vi "creat tasks.vi"   [LabVIEW 2017]
uses:
  <vilib>/DAQmx/create/channels.llb/DAQmx Create Channel (TEDS-AI-Current-Basic).vi
  <vilib>/DAQmx/create/channels.llb/DAQmx Create Channel (AI-Current-Basic).vi
  <resource>/objmgr/daqmx.rc
  <vilib>/DAQmx/create/channels.llb/DAQmx Create Channel (AI-Voltage-Basic).vi
  <vilib>/DAQmx/create/channels.llb/DAQmx Create Channel (AI-Temperature-RTD).vi
  <vilib>/DAQmx/create/channels.llb/DAQmx Create Channel (AI-Temperature-Thermocouple).vi
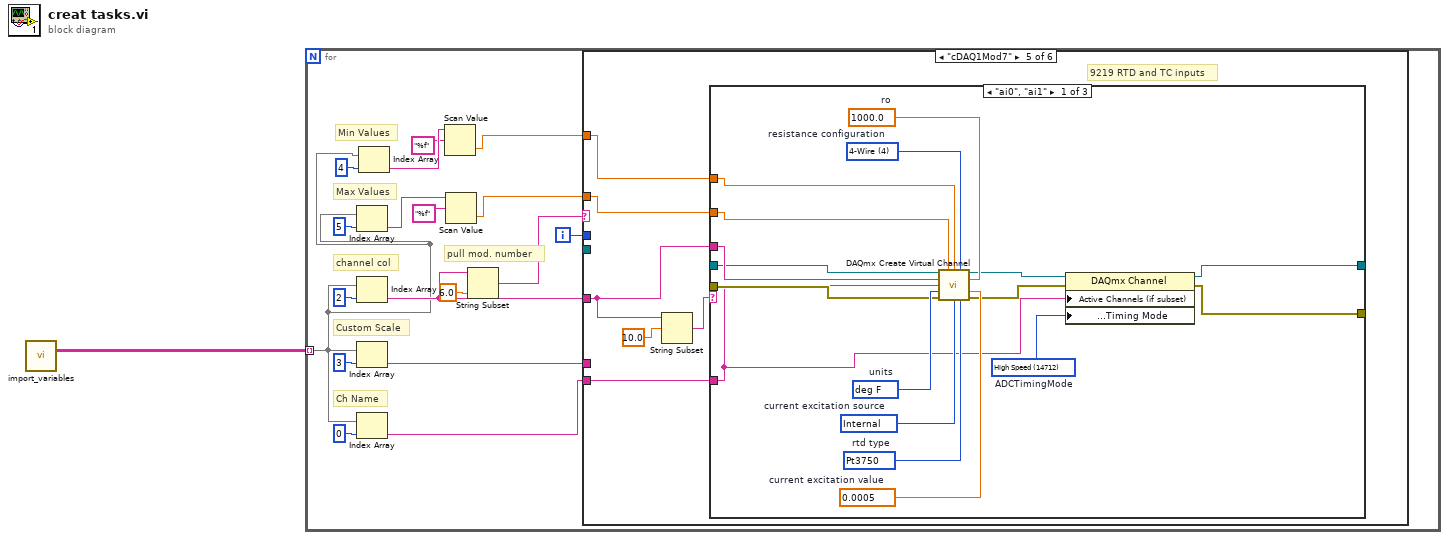
[diagram p0: block diagram]
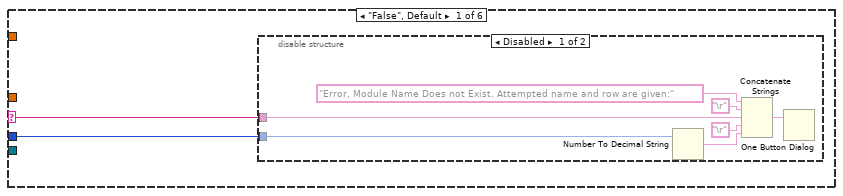
[diagram p2: hidden frame]
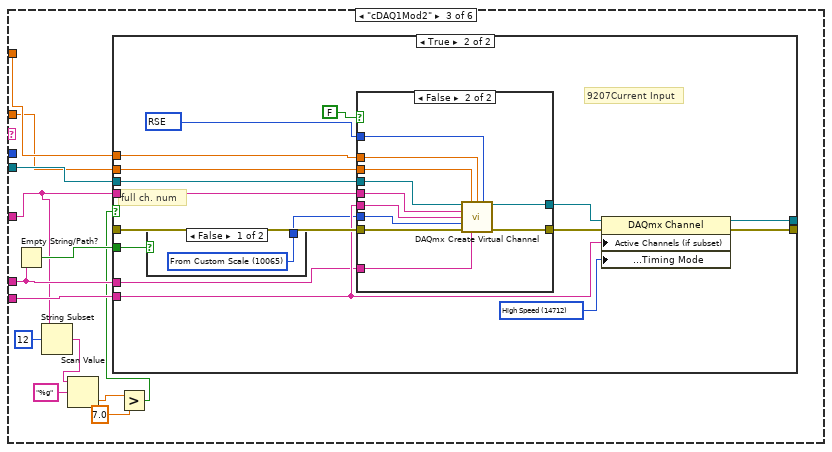
[diagram p5: hidden frame]
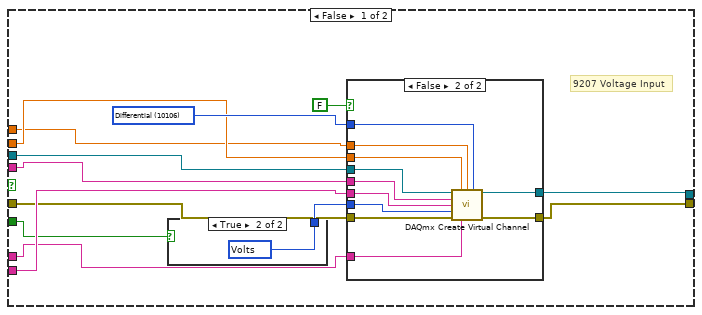
[diagram p6: hidden frame]
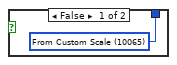
[diagram p7: hidden frame]
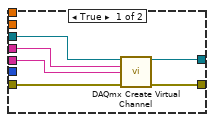
[diagram p8: hidden frame]
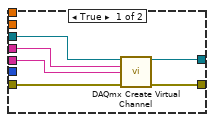
[diagram p9: hidden frame]
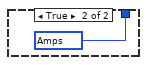
[diagram p10: hidden frame]
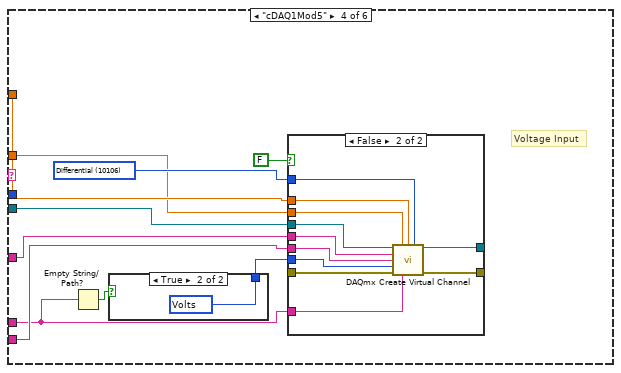
[diagram p11: hidden frame]
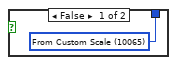
[diagram p12: hidden frame]
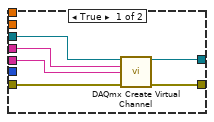
[diagram p13: hidden frame]
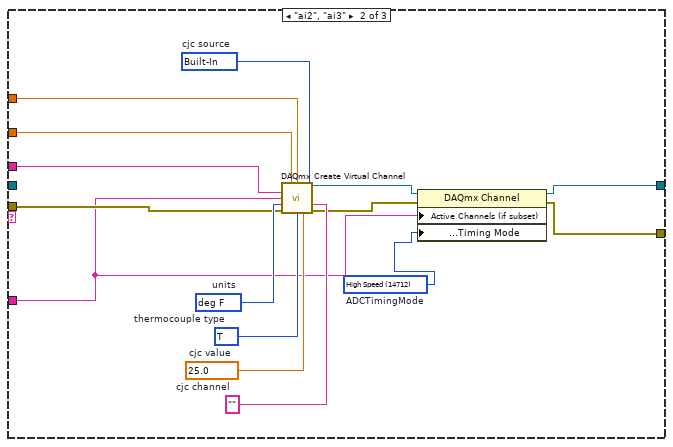
[diagram p14: hidden frame]
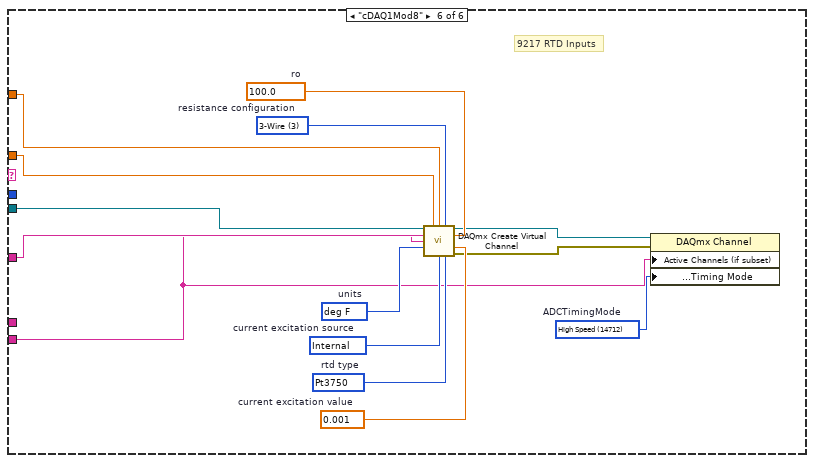
[diagram p16: hidden frame]
diagram:
  n1 = call "import_variables.vi"() -> ("String Array From File"=w1:string[][])  [unwired: 10 in, 1 out]
  n2 = for {
    tunnel: w1 -> [w8] mode=indexing
    i -> [w12]
    # "Max Values"
    # "Min Values"
    # "Custom Scale"
    # "Ch Name"
    # "channel col"
    # "pull mod. number"
    n3 = Index Array(array=w8, index=5) -> (element=w3:string)
    n4 = Index Array(array=w8, index=2) -> (element=w11:string)
    n5 = Index Array(array=w8, index=3) -> (element=w13:string)
    n6 = Index Array(array=w8, index=0) -> (element=w15:string)
    n7 = Index Array(array=w8, index=4) -> (element=w7:string)
    n8 = Scan Value(string=w7, format string="%f") -> (value=w6:dbl)  [unwired: 1 in, 1 out]
    n9 = Scan Value(string=w3, format string="%f") -> (value=w2:dbl)  [unwired: 1 in, 1 out]
    n10 = String Subset(string=w11, length (rest)=6.0) -> (substring=w17:string)  [unwired: 1 in]
    n11 = case shown="\"cDAQ1Mod7\"" w17 {
      selector: w17 -> [w21 _ _ _ _ _]
      tunnel: w15 -> [_ _ w42 w123 w150 w188]
      tunnel: _ -> [w22 _ w44 w122 _ w194]
      tunnel: w13 -> [_ _ w40 w116 _ _]
      tunnel: w12 -> [w20 _ _ _ _ _]
      tunnel: w11 -> [_ _ w35 w117 w147 w197]
      tunnel: w6 -> [_ _ w38 w113 w149 w187]
      tunnel: w2 -> [_ _ w37 w112 w148 w196]
      frame "False", Default {
        n12 = disable-structure shown="Disabled" {
          disable-tunnel: w21 -> [w27 _]
          disable-tunnel: w20 -> [w25 _]
          frame Disabled {
            n13 = Number To Decimal String(number=w25) -> (decimal integer string=w24:string)  [unwired: 1 in]
            n14 = Concatenate Strings("Error, Module Name Does not Exist. Attempted name and row are given:", "\r", w27, "\r", w24) -> (w23:string)
            n15 = One Button Dialog(message=w23) -> ()  [unwired: 1 in, 1 out]
          }
          frame Enabled {
          }
        }
      }
      frame "NI9208" {
      }
      frame "cDAQ1Mod2" {
        n16 = Empty String/Path?(string/path=w40) -> (empty?=w39:bool)
        n17 = String Subset(string=w35, offset (0)=12) -> (substring=w34:string)  [unwired: 1 in]
        n18 = Scan Value(string=w34, format string="%g") -> (value=w32:dbl)  [unwired: 1 in, 1 out]
        n19 = Greater?(x=w32, y=7.0) -> (0:w30:bool)
        n20 = case shown="True" w30 {
          tunnel: w44 -> [w52 w91]
          tunnel: [w49 w90] -> w43
          tunnel: w42 -> [w50 w89]
          tunnel: [w46 w86] -> w41
          tunnel: [w45 w85] -> _
          tunnel: w35 -> [w51 w82]
          tunnel: w40 -> [w48 w80]
          tunnel: w39 -> [w47 w79]
          tunnel: w38 -> [w53 w78]
          tunnel: w37 -> [w54 w77]
          frame False {
            w56 = 10106 items=["default"=-1, "RSE"=10083, "NRSE"=10078, "Differential"=10106, "Pseudodifferential"=12529] ("input terminal configuration")
            # "9207 Voltage Input"
            n21 = case shown="True" w47 {
              tunnel: [w58 w59] -> w55
              frame False {
                w58 = 10065 items=["Amps"=10342, "From TEDS"=12516, "From Custom Scale"=10065] ("units")
              }
              frame True {
                w59 = 10348 items=["Volts"=10348, "From TEDS"=12516, "From Custom Scale"=10065] ("units")
              }
            }
            n22 = case shown="False" FALSE {
              tunnel: [w65 w76] -> w46
              tunnel: [w64 w75] -> w45
              tunnel: w50 -> [w63 w73]
              tunnel: w52 -> [w62 w74]
              tunnel: w49 -> [w61 w72]
              tunnel: w51 -> [w60 w71]
              tunnel: w48 -> [_ w70]
              tunnel: w55 -> [_ w69]
              tunnel: w56 -> [_ w68]
              tunnel: w54 -> [_ w67]
              tunnel: w53 -> [_ w66]
              frame True {
                n23 = call-poly <vilib>:"DAQmx Create Virtual Channel.vi"("task in"=w62, "physical channels"=w60, "name to assign"=w63, "error in"=w61) -> ("task out"=w65:refnum<k21>, "error out"=w64:errorcluster)  [unwired: 10 in]
              }
              frame False {
                n24 = call-poly <vilib>:"DAQmx Create Virtual Channel.vi"("task in"=w74, "maximum value"=w67, "minimum value"=w66, "input terminal configuration"=w68, "physical channels"=w71, "name to assign"=w73, "units"=w69, "error in"=w72, "custom scale name"=w70) -> ("task out"=w76:refnum<k21>, "error out"=w75:errorcluster)  [unwired: 5 in]
              }
            }
          }
          frame True {
            w81 = 14712 items=["High Resolution"=10195, "High Speed"=14712, "Best 50 Hz Rejection"=14713, "Best 60 Hz Rejection"=14714] ("AI.ADCTimingMode")
            w84 = 10083 items=["default"=-1, "RSE"=10083, "NRSE"=10078, "Differential"=10106, "Pseudodifferential"=12529] ("input terminal configuration")
            # "full ch. num"
            # "9207Current Input"
            n25 = case shown="False" w79 {
              tunnel: [w110 w111] -> w83
              frame False {
                w110 = 10065 items=["Amps"=10342, "From TEDS"=12516, "From Custom Scale"=10065] ("units")
              }
              frame True {
                w111 = 10342 items=["Amps"=10342, "From TEDS"=12516, "From Custom Scale"=10065] ("units")
              }
            }
            n26 = case shown="False" FALSE {
              tunnel: [w98 w109] -> w88
              tunnel: [w97 w108] -> w87
              tunnel: w89 -> [w96 w106]
              tunnel: w91 -> [w95 w107]
              tunnel: w90 -> [w94 w105]
              tunnel: w82 -> [w93 w104]
              tunnel: w80 -> [_ w103]
              tunnel: w83 -> [_ w102]
              tunnel: w77 -> [_ w101]
              tunnel: w78 -> [_ w100]
              tunnel: w84 -> [_ w99]
              frame True {
                n27 = call-poly <vilib>:"DAQmx Create Virtual Channel.vi"("task in"=w95, "physical channels"=w93, "name to assign"=w96, "error in"=w94) -> ("task out"=w98:refnum<k21>, "error out"=w97:errorcluster)  [unwired: 10 in]
              }
              frame False {
                n28 = call-poly <vilib>:"DAQmx Create Virtual Channel.vi"("task in"=w107, "maximum value"=w101, "minimum value"=w100, "input terminal configuration"=w99, "physical channels"=w104, "name to assign"=w106, "units"=w102, "error in"=w105, "custom scale name"=w103) -> ("task out"=w109:refnum<k21>, "error out"=w108:errorcluster)  [unwired: 5 in]
              }
            }
            n29 = property class="DAQmx Channel"(reference=w88, error in=w87, "Active Channels (if subset)"=w89, "Analog Input:General Properties:Digitizer/ADC:Timing Mode"=w81) -> (reference out=w86:refnum<k21>, error out=w85:errorcluster)
          }
        }
      }
      frame "cDAQ1Mod5" {
        w120 = 10106 items=["default"=-1, "RSE"=10083, "NRSE"=10078, "Differential"=10106, "Pseudodifferential"=12529] ("input terminal configuration")
        # "Voltage Input"
        n30 = Empty String/Path?(string/path=w116) -> (empty?=w115:bool)
        n31 = case shown="True" w115 {
          tunnel: [w125 w126] -> w114
          frame False {
            w125 = 10065 items=["Amps"=10342, "From TEDS"=12516, "From Custom Scale"=10065] ("units")
          }
          frame True {
            w126 = 10348 items=["Volts"=10348, "From TEDS"=12516, "From Custom Scale"=10065] ("units")
          }
        }
        n32 = case shown="False" FALSE {
          tunnel: [w132 w143] -> w119
          tunnel: [w131 w142] -> w118
          tunnel: w123 -> [w130 w140]
          tunnel: w122 -> [w129 w141]
          tunnel: [w128 w139] -> w121
          tunnel: w117 -> [w127 w138]
          tunnel: w116 -> [_ w137]
          tunnel: w114 -> [_ w136]
          tunnel: w120 -> [_ w135]
          tunnel: w112 -> [_ w134]
          tunnel: w113 -> [_ w133]
          frame True {
            n33 = call-poly <vilib>:"DAQmx Create Virtual Channel.vi"("task in"=w129, "physical channels"=w127, "name to assign"=w130, "error in"=w128) -> ("task out"=w132:refnum<k21>, "error out"=w131:errorcluster)  [unwired: 10 in]
          }
          frame False {
            n34 = call-poly <vilib>:"DAQmx Create Virtual Channel.vi"("task in"=w141, "maximum value"=w134, "minimum value"=w133, "input terminal configuration"=w135, "physical channels"=w138, "name to assign"=w140, "units"=w136, "error in"=w139, "custom scale name"=w137) -> ("task out"=w143:refnum<k21>, "error out"=w142:errorcluster)  [unwired: 5 in]
          }
        }
      }
      frame "cDAQ1Mod7" {
        # "9219 RTD and TC inputs"
        n35 = String Subset(string=w147, offset (0)=10.0) -> (substring=w151:string)  [unwired: 1 in]
        n36 = case shown="\"ai0\", \"ai1\"" w151 {
          tunnel: w150 -> [w155 w172 _]
          tunnel: w149 -> [w160 w179 _]
          tunnel: w148 -> [w159 w178 _]
          tunnel: w147 -> [w163 w177 _]
          tunnel: _ -> [w161 _ w186]
          tunnel: [w162 w176 w185] -> w146
          tunnel: [w154 w171 w186] -> w145
          tunnel: [w153 w170 w185] -> w144
          frame "ai0", "ai1" {
            w156 = 14712 items=["High Resolution"=10195, "High Speed"=14712, "Best 50 Hz Rejection"=14713, "Best 60 Hz Rejection"=14714]  # ADCTimingMode
            w164 = 12481 items=["Pt3750"=12481, "Pt3851"=10071, "Pt3911"=12482, "Pt3916"=10069, "Pt3920"=10053, "Pt3928"=12483, "Custom"=10137]  # rtd type
            w165 = 0.0005  # current excitation value
            w166 = 1000.0  # ro
            w167 = 4 items=["2-Wire"=2, "3-Wire"=3, "4-Wire"=4]  # resistance configuration
            w168 = 10200 items=["Internal"=10200, "External"=10167, "None"=10230]  # current excitation source
            w169 = 10144 items=["deg C"=10143, "deg F"=10144, "Kelvins"=10325, "deg R"=10145, "From Custom Scale"=10065]  # units
            n37 = call-poly <vilib>:"DAQmx Create Virtual Channel.vi"("task in"=w161, "maximum value"=w159, "minimum value"=w160, "resistance configuration"=w167, "physical channels"=w163, "r0"=w166, "name to assign"=w155, "units"=w169, "current excitation value"=w165, "error in"=w162, "current excitation source"=w168, "rtd type"=w164) -> ("task out"=w158:refnum<k21>, "error out"=w157:errorcluster)  [unwired: 2 in]
            n38 = property class="DAQmx Channel"(reference=w158, error in=w157, "Active Channels (if subset)"=w155, "Analog Input:General Properties:Digitizer/ADC:Timing Mode"=w156) -> (reference out=w154:refnum<k21>, error out=w153:errorcluster)
          }
          frame "ai2", "ai3" {
            w175 = 14712 items=["High Resolution"=10195, "High Speed"=14712, "Best 50 Hz Rejection"=14713, "Best 60 Hz Rejection"=14714]  # ADCTimingMode
            w180 = 10200 items=["Built-In"=10200, "Constant Value"=10116, "Channel"=10113]  # cjc source
            w181 = ""  # cjc channel
            w182 = 25.0  # cjc value
            w183 = 10086 items=["J"=10072, "K"=10073, "N"=10077, "R"=10082, "S"=10085, "T"=10086, "B"=10047, "E"=10055]  # thermocouple type
            w184 = 10144 items=["deg C"=10143, "deg F"=10144, "Kelvins"=10325, "deg R"=10145, "From Custom Scale"=10065]  # units
            n39 = call-poly <vilib>:"DAQmx Create Virtual Channel.vi"("maximum value"=w178, "minimum value"=w179, "physical channels"=w177, "cjc source"=w180, "name to assign"=w172, "units"=w184, "cjc channel"=w181, "error in"=w176, "thermocouple type"=w183, "cjc value"=w182) -> ("task out"=w174:refnum<k21>, "error out"=w173:errorcluster)  [unwired: 4 in]
            n40 = property class="DAQmx Channel"(reference=w174, error in=w173, "Active Channels (if subset)"=w172, "Analog Input:General Properties:Digitizer/ADC:Timing Mode"=w175) -> (reference out=w171:refnum<k21>, error out=w170:errorcluster)
          }
          frame "false", Default {
          }
        }
      }
      frame "cDAQ1Mod8" {
        w193 = 14712 items=["High Resolution"=10195, "High Speed"=14712, "Best 50 Hz Rejection"=14713, "Best 60 Hz Rejection"=14714]  # ADCTimingMode
        w198 = 12481 items=["Pt3750"=12481, "Pt3851"=10071, "Pt3911"=12482, "Pt3916"=10069, "Pt3920"=10053, "Pt3928"=12483, "Custom"=10137]  # rtd type
        w199 = 0.001  # current excitation value
        w200 = 100.0  # ro
        w201 = 3 items=["2-Wire"=2, "3-Wire"=3, "4-Wire"=4]  # resistance configuration
        w202 = 10200 items=["Internal"=10200, "External"=10167, "None"=10230]  # current excitation source
        w203 = 10144 items=["deg C"=10143, "deg F"=10144, "Kelvins"=10325, "deg R"=10145, "From Custom Scale"=10065]  # units
        # "9217 RTD Inputs"
        n41 = call-poly <vilib>:"DAQmx Create Virtual Channel.vi"("task in"=w194, "maximum value"=w196, "minimum value"=w187, "resistance configuration"=w201, "physical channels"=w197, "r0"=w200, "name to assign"=w188, "units"=w203, "current excitation value"=w199, "current excitation source"=w202, "rtd type"=w198) -> ("task out"=w192:refnum<k21>, "error in"=w195:errorcluster, "error out"=w191:errorcluster)  [unwired: 2 in]
        n42 = property class="DAQmx Channel"(reference=w192, error in=w191, "Active Channels (if subset)"=w188, "Analog Input:General Properties:Digitizer/ADC:Timing Mode"=w193) -> (reference out=w190:refnum<k21>, error out=w189:errorcluster)
      }
    }
  }
